vi "LVClass_CorrectionDataManager SetMicrolensesFocalLength.vi"(0 "CorrectionDataManager in":refnum<class "CorrectionDataManager.lvclass">, 5 "MicrolensesFocalLength":sgl, 11 "error in (no error)":errorcluster) -> (4 "CorrectionDataManager out":refnum<class "CorrectionDataManager.lvclass">, 15 "error out":errorcluster)   [LabVIEW 2020, in "CorrectionDataManager.lvclass"]
doc: "Micro lenses focal length setter. .\n\n<B>corrdata_managerIn</B> : CorrDataManager object.\n<B>corrdata_managerOut</B> : CorrDataManager object.\n<B>microlenses_focal_length_um</B> : Micro lenses focal length (um)."
uses:
  CorrectionDataManager.lvclass
  CorrectionDataManager.lvclass/CorrectionDataManager.ctl
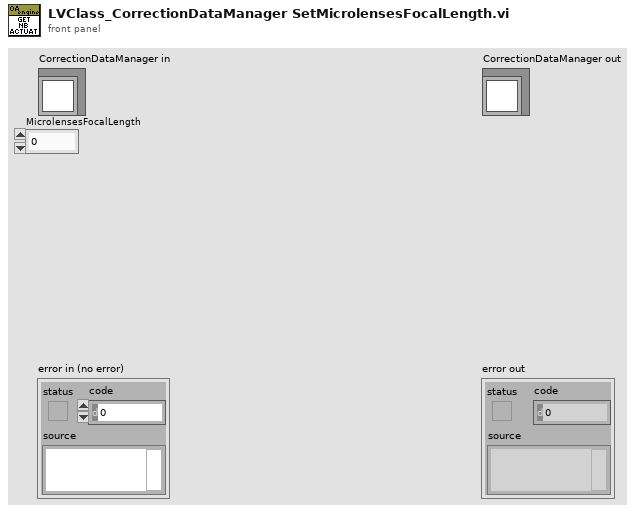
[diagram p1: front panel]
types:
  T1 = typedef "ClassID.ctl" = i64
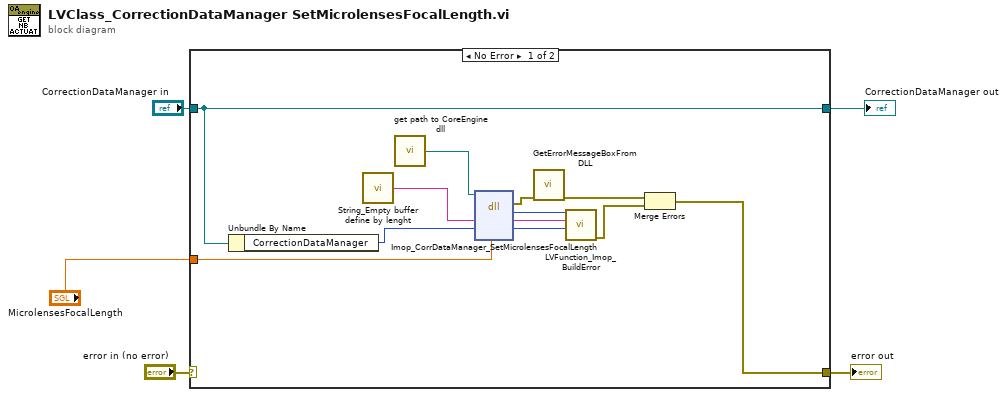
[diagram p0: block diagram]
diagram:
  n1 = case shown="No Error" "error in (no error)" {
    selector: "error in (no error)" -> [_ w19]
    tunnel: [w10 w19] -> w3
    tunnel: [w9 w18] -> w2
    tunnel: "CorrectionDataManager in" -> [w9 w18]
    tunnel: "MicrolensesFocalLength" -> [w7 _]
    frame No Error {
      n2 = Unbundle By Name(w9) -> ("CorrectionDataManager"=w8:T1)
      n3 = call "String_Empty buffer define by lenght.vi"() -> ("Empty buffer"=w15:string)  [unwired: 1 in]
      n4 = call "get path to CoreEngine dll.vi"() -> ("path to wavekit library"=w14:path)  [unwired: 14 in, 1 out]
      n5 = dll-call lib="D:/soft/HASO_v3/SVN_trunk/ImOpCoreEngine4_LV2011/DLLs/c_interface_vc100.dll" fn="Imop_CorrDataManager_SetMicrolensesFocalLength"(path in=w14, "message"=w15, "WavefrontCorrection"=w8, "MicrolensesFocalLength"=w7) -> (error out=w13:errorcluster, "return type"=w17:i32, "message"=w16:string, "WavefrontCorrection"=w6:i64)  [unwired: 3 in, 1 out]
      n6 = call "GetErrorMessageBoxFromDLL.vi"("error IN"=w13) -> ("error OUT"=w12:errorcluster)  [unwired: 10 in]
      n7 = call "LVFunction_Imop_BuildError.vi"("code"=w17, "String to Prepend to source (\"\")"=w16, "Adresse"=w6) -> ("error out"=w11:errorcluster)  [unwired: 12 in]
      n8 = Merge Errors(w12, w11) -> (w10:errorcluster)
    }
    frame Error {
    }
  }
  "error out" <- w3
  "CorrectionDataManager out" <- w2
